vi "Finish.vi"   [LabVIEW 2015]
doc: "This VI is called just before exiting. It is expected to close I/O refnum, save collected data, etc."
uses:
  <vilib>/Rock Robotics/WPI/Utilities/WPI_GetSetVariantRefNum.vi
types:
  T1 = typedef "WPI_SolenoidDevRef.ctl" = cluster{"DevStatus":errorcluster, "Pneumatics Control Module":u8, "Forward Solenoid Channel":T2, "Reverse Solenoid Channel":T2}
  T2 = typedef "WPI_SolenoidChannel.ctl" = enum8{"Solenoid 0", "Solenoid 1", "Solenoid 2", "Solenoid 3", "Solenoid 4", "Solenoid 5", "Solenoid 6", "Solenoid 7", "Invalid"}
  T3 = typedef "WPI_GyroDevRef.ctl" = cluster{"DevStatus":errorcluster, "Analog Channel":T4, "Offset":dbl, "Gain (VoltsPerDegree/Second)":dbl, "Gyro Type":enum16{"Analog", "XRS450"}, "Handle":i32, "SPI Bus":T5, "Device Found":bool, "Sample Rate":dbl, "Calibrate On Open":bool}
  T4 = typedef "FPGA_AIChannel.ctl" = enum8{"AI 0", "AI 1", "AI 2", "AI 3", "AI MXP 0", "AI MXP 1", "AI MXP 2", "AI MXP 3", "Invalid"}
  T5 = typedef "spi_bus.ctl" = enum16{"SPI On-Board, CS0", "SPI On-Board, CS1", "SPI On-Board, CS2", "SPI On-Board, CS3", "SPI MXP", "Invalid"}
  T6 = typedef "WPI_PotentiometerDevRef.ctl" = cluster{"DevStatus":errorcluster, "Analog Channel":T4, "Invert Output":bool}
  T7 = typedef "WPI_RobotDriveDevRef.ctl" = cluster{"DevStatus":errorcluster, "Motors[]":T8[], "Square Inputs":bool, "Max Output":dbl}
  T8 = typedef "WPI_MotorControlDeviceRef.ctl" = cluster{"DeviceStatus":errorcluster, "Type":T9, "PWM":cluster{"PWM Channel":T10, "DeadBand":T11}, "CAN":cluster{"Device Number":u8, "Control Mode":T12, "Semaphore":T13, "Max Vout":dbl, "TalonSRX Control Mode":T14}, "Invert":bool}
  T9 = typedef "WPI_MotorControlType.ctl" = enum16{"PWM", "CAN", "CANTalonSRX"}
  T10 = typedef "FPGA_DIOPWMChannel.ctl" = enum8{"PWM 0", "PWM 1", "PWM 2", "PWM 3", "PWM 4", "PWM 5", "PWM 6", "PWM 7", "PWM 8", "PWM 9", "PWM MXP 0", "PWM MXP 1", "PWM MXP 2", "PWM MXP 3", "PWM MXP 4", "PWM MXP 5", "PWM MXP 6", "PWM MXP 7", "PWM MXP 8", "PWM MXP 9", "Invalid"}
  T11 = typedef "WPI_PWMDeadband.ctl" = cluster{"Name":string, "maxPositivePwm":i32, "minPositivePwm":i32, "centerPwm":i32, "maxNegativePwm":i32, "minNegativePwm":i32, "angularRange":u16}
  T12 = typedef "WPI_CANJaguar_ControlMode.ctl" = enum8{"Percent VBus", "Current", "Speed", "Position", "Voltage"}
  T13 = typedef "Semaphore RefNum" = refnum<k1>
  T14 = typedef "WPI_CANTalonSRX_APIControlMode.ctl" = enum8{"Percent VBus", "Speed", "Position", "Slave", "Unchanged / Invalid", "Voltage Compensation", "Current", "Motion Profile"}
  T15 = typedef "WPI_JoystickDevRef.ctl" = cluster{"Device":T16}
  T16 = typedef "WPI_JoystickDeviceEnum.ctl" = enum16{"USB 0", "USB 1", "USB 2", "USB 3", "USB 4", "USB 5"}
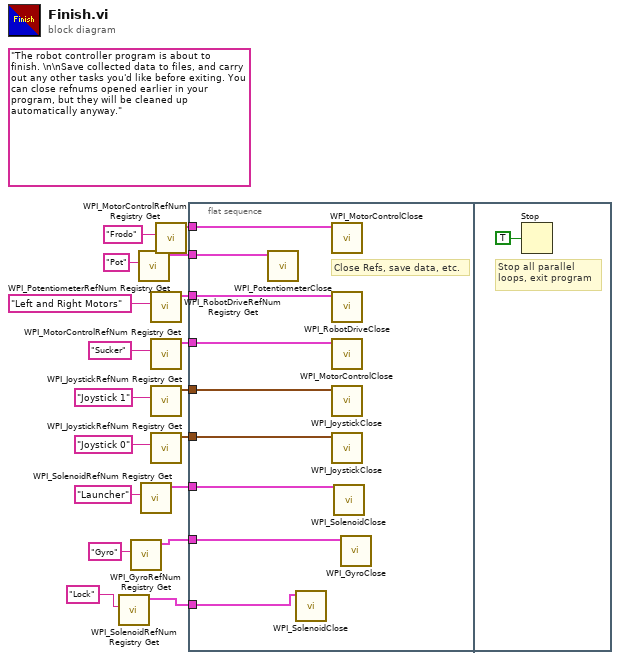
[diagram p0: block diagram]
diagram:
  (unwired) "The robot controller program is about to finish. \n\nSave collected data to files, and carry out any other tasks you'd like before exiting. You can close refnums opened earlier in your program, but they will be cleaned up automatically anyway."
  n1 = call <vilib>:"WPI_SolenoidRefNum Registry Get.vi"("refnum name"="Lock") -> ("SolenoidDevRef"=w4:T1)  [unwired: 9 in, 1 out]
  n2 = call <vilib>:"WPI_GyroRefNum Registry Get.vi"("refnum name"="Gyro") -> ("GyroDevRef"=w7:T3)  [unwired: 9 in, 1 out]
  n3 = call <vilib>:"WPI_PotentiometerRefNum Registry Get.vi"("refnum name"="Pot") -> ("PotDevRef"=w2:T6)  [unwired: 9 in, 1 out]
  n4 = call <vilib>:"WPI_SolenoidRefNum Registry Get.vi"("refnum name"="Launcher") -> ("SolenoidDevRef"=w9:T1)  [unwired: 9 in, 1 out]
  n5 = call <vilib>:"WPI_RobotDriveRefNum Registry Get.vi"("refnum name"="Left and Right Motors") -> ("RobotDriveDevRef"=w16:T7)  [unwired: 1 in, 9 out]
  n6 = call <vilib>:"WPI_MotorControlRefNum Registry Get.vi"("refnum name"="Sucker") -> ("MotorControlDevRef"=w14:T8)  [unwired: 9 in, 1 out]
  n7 = call <vilib>:"WPI_JoystickRefNum Registry Get.vi"("refnum name"="Joystick 1") -> ("JoystickDevRef"=w10:T15)  [unwired: 9 in, 1 out]
  n8 = call <vilib>:"WPI_JoystickRefNum Registry Get.vi"("refnum name"="Joystick 0") -> ("JoystickDevRef"=w15:T15)  [unwired: 1 in, 9 out]
  n9 = call <vilib>:"WPI_MotorControlRefNum Registry Get.vi"("refnum name"="Frodo") -> ("MotorControlDevRef"=w13:T8)  [unwired: 9 in, 1 out]
  n10 = flat-sequence {
    tunnel: w16 -> [w27]
    tunnel: w15 -> [w26]
    tunnel: w14 -> [w25]
    tunnel: w13 -> [w24]
    tunnel: w10 -> [w23]
    tunnel: w9 -> [w22]
    tunnel: w7 -> [w21]
    tunnel: w4 -> [w20]
    tunnel: w2 -> [w19]
    frame #0 {
      # "Close Refs, save data, etc."
      n11 = call <vilib>:"WPI_PotentiometerClose.vi"("PotDevRef"=w19) -> ()  [unwired: 10 in, 1 out]
      n12 = call <vilib>:"WPI_SolenoidClose.vi"("SolenoidDevRef"=w20) -> ()  [unwired: 10 in, 1 out]
      n13 = call <vilib>:"WPI_MotorControlClose.vi"("MotorControlDevRef"=w24) -> ()  [unwired: 10 in, 1 out]
      n14 = call <vilib>:"WPI_RobotDriveClose.vi"("RobotDriveDevRef"=w27) -> ()  [unwired: 1 in, 10 out]
      n15 = call <vilib>:"WPI_MotorControlClose.vi"("MotorControlDevRef"=w25) -> ()  [unwired: 10 in, 1 out]
      n16 = call <vilib>:"WPI_JoystickClose.vi"("JoystickDevRef"=w23) -> ()  [unwired: 11 in]
      n17 = call <vilib>:"WPI_JoystickClose.vi"("JoystickDevRef"=w26) -> ()  [unwired: 11 out]
      n18 = call <vilib>:"WPI_SolenoidClose.vi"("SolenoidDevRef"=w22) -> ()  [unwired: 10 in, 1 out]
      n19 = call <vilib>:"WPI_GyroClose.vi"("GyroDevRef"=w21) -> ()  [unwired: 10 in, 1 out]
    }
    frame #1 {
      # "Stop all parallel\nloops, exit program"
      n20 = Stop(stop? (T)=TRUE ("Quit")) -> ()
    }
  }
